vi "Example Type Cast 1.vi"() -> ()   [LabVIEW 2014]
panel:
  out "case2":sgl
  out "case4":u8[](array[numeric])
  out "case3":u8[](array[numeric])
  out "case1":u8
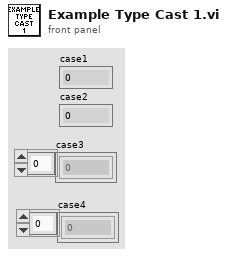
[diagram p1: front panel]
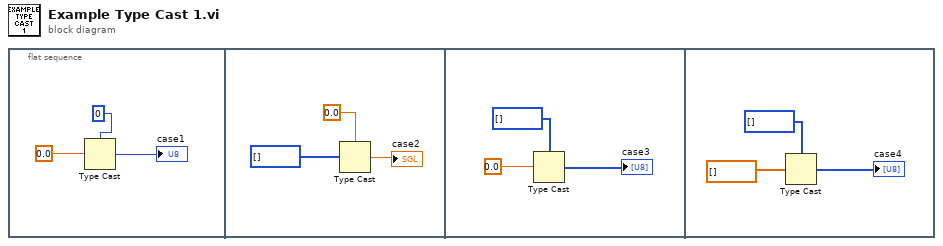
[diagram p0: block diagram]
diagram:
  n1 = flat-sequence {
    frame #0 {
      n2 = Type Cast(type=u8 0, x=sgl 0.0) -> (*(type *) &x=→"case1":u8)
    }
    frame #1 {
      n3 = Type Cast(type=sgl 0.0, x=u8[] []) -> (*(type *) &x=→"case2":sgl)
    }
    frame #2 {
      n4 = Type Cast(type=u8[] [], x=sgl 0.0) -> (*(type *) &x=→"case3":u8[])
    }
    frame #3 {
      n5 = Type Cast(type=u8[] [], x=sgl[] []) -> (*(type *) &x=→"case4":u8[])
    }
  }
